vi "Advance past Number.vi"(7 "JSON":string, 9 "Offset (0)":i32, 11 "Parser State in":T2=enum."Number/Other") -> (1 "Offset past match":i32, 2 "LabVIEW Extension (NaN, Infinity)":bool, 3 "Parser State":T2, 4 "JSON Value Type":T1, 6 "Value start out":i32)   [LabVIEW 2020, in "JSONtext.lvlib"]
uses:
  <vilib>/JDP Science/JSONtext/JSONtext.lvlib
  <vilib>/JDP Science/JSONtext/Parsing/Parsing State.ctl
  <vilib>/JDP Science/JSONtext/JSON Value Type.ctl
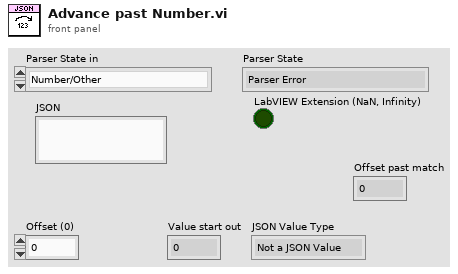
[diagram p1: front panel]
types:
  T1 = typedef "JSONtext.lvlib/JSON Value Type.ctl" = enum16{"Not a JSON Value", "JSON Object", "JSON Array", "String", "Number", "true", "false", "null"}
  T2 = typedef "JSONtext.lvlib/Parsing State.ctl" = enum16{"Parser Error", "Object", "Array", "String", "Number/Other", "Leading Whitespace", "Object end", "Array end", "Value end"}
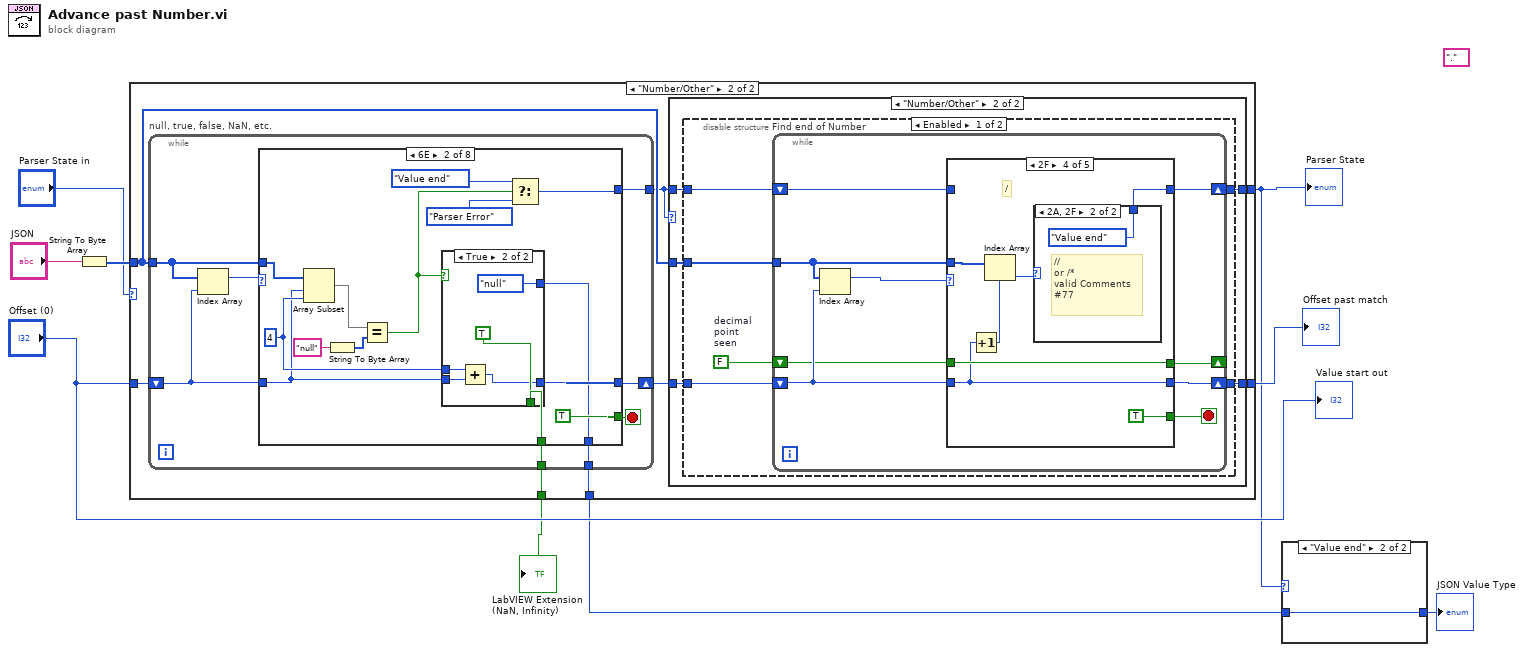
[diagram p0: block diagram]
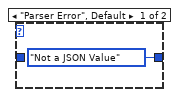
[diagram p2: hidden frame]
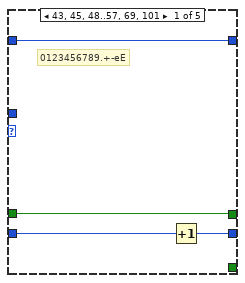
[diagram p5: hidden frame]
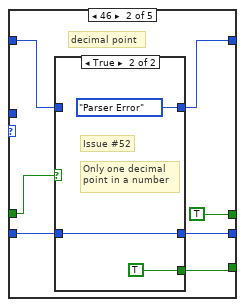
[diagram p6: hidden frame]
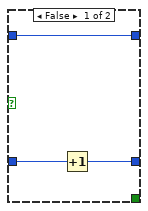
[diagram p7: hidden frame]
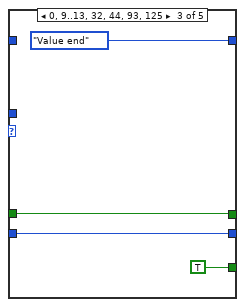
[diagram p8: hidden frame]
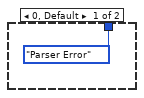
[diagram p9: hidden frame]
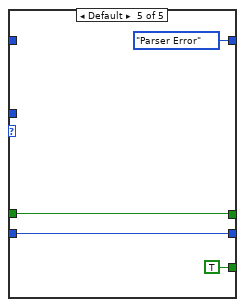
[diagram p10: hidden frame]
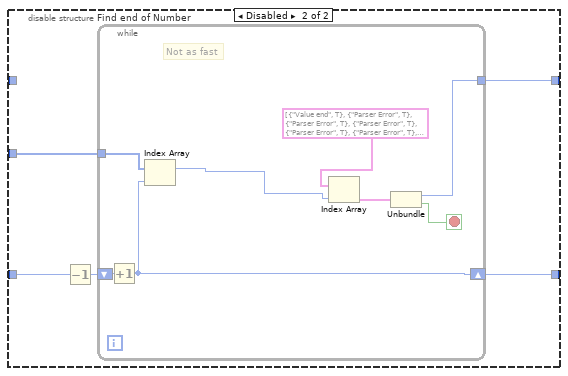
[diagram p11: hidden frame]
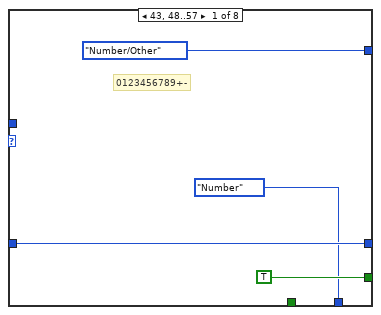
[diagram p12: hidden frame]
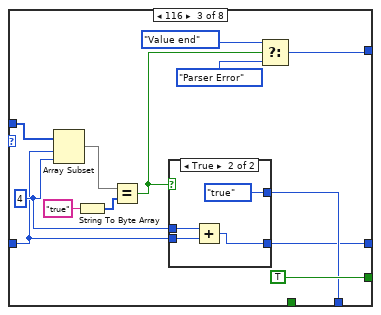
[diagram p14: hidden frame]
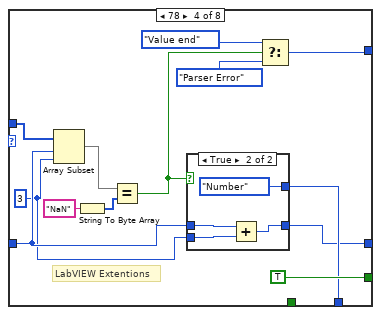
[diagram p16: hidden frame]
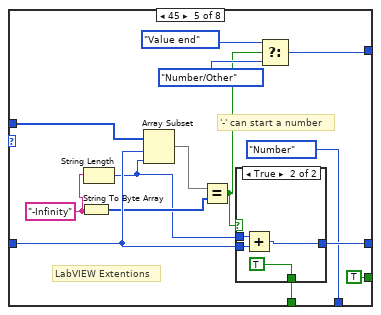
[diagram p18: hidden frame]
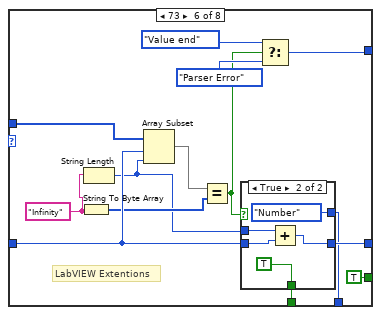
[diagram p20: hidden frame]
diagram:
  (unwired) "."
  n1 = String To Byte Array(string="JSON") -> (unsigned byte array=w6:u8[])
  n2 = case shown="\"Number/Other\"" "Parser State in" {
    tunnel: [_ w18] -> w4
    tunnel: [w10 w17] -> w9
    tunnel: w6 -> [_ w15]
    tunnel: "Offset (0)" -> [w10 w13]
    tunnel: [_ w12] -> w3
    tunnel: [_ w11] -> w1
    frame "Parser Error", Default {
    }
    frame "Number/Other" {
      n3 = while "null, true, false, NaN, etc." {
        tunnel: w15 -> [w94]
        shift-right: [w90] -> w16
        shift-left: w13 -> [w91]
        tunnel: [w93] -> w14
        tunnel: [w89] -> w12
        tunnel: [w88] -> w11
        stop <- w92 stop-if-true
        n4 = Index Array(array=w94, index=w91) -> (element=w95:u8)
        n5 = case shown="6E" w95 {
          tunnel: w94 -> [_ w112 w131 w149 w169 w188 w206 _]
          tunnel: [Parsing_State."Number/Other" w109 w128 w146 w167 w186 w203 Parsing_State."Parser Error"] -> w93
          tunnel: [TRUE TRUE TRUE TRUE TRUE TRUE TRUE TRUE] -> w92
          tunnel: w91 -> [w97 w101 w121 w140 w163 w182 w199 w212]
          tunnel: [w97 w100 w120 w138 w162 w181 w197 w212] -> w90
          tunnel: [JSON_Value_Type."Number" w104 w123 w141 JSON_Value_Type."Number" w176 w195 JSON_Value_Type."Not a JSON Value"] -> w89
          tunnel: [_ w103 _ _ w156 w175 _ _] -> w88
          frame 43, 48..57 {
            # "0123456789+-"
          }
          frame 110 {
            w102 = 4 ("length")
            n6 = Array Subset(array=w112, index=w101, length=w102) -> (w110:u8[])
            n7 = String To Byte Array(string="null") -> (unsigned byte array=w111:u8[])
            n8 = Equal?(x=w110, y=w111) -> (x = y?=w105:bool)
            n9 = case shown="True" w105 {
              tunnel: [_ JSON_Value_Type."null"] -> w104
              tunnel: [_ TRUE] -> w103
              tunnel: w102 -> [_ w117]
              tunnel: w101 -> [w114 w116]
              tunnel: [w114 w115] -> w100
              frame False {
              }
              frame True {
                n10 = Add(x=w117, y=w116) -> (x+y=w115:i32)
              }
            }
            n11 = Select(t=Parsing_State."Value end", s=w105, f=Parsing_State."Parser Error") -> (s? t:f=w109:T2)
          }
          frame 116 {
            w122 = 4 ("length")
            n12 = Array Subset(array=w131, index=w121, length=w122) -> (w129:u8[])
            n13 = String To Byte Array(string="true") -> (unsigned byte array=w130:u8[])
            n14 = Equal?(x=w129, y=w130) -> (x = y?=w124:bool)
            n15 = case shown="True" w124 {
              tunnel: [_ JSON_Value_Type."true"] -> w123
              tunnel: w122 -> [_ w136]
              tunnel: w121 -> [w133 w135]
              tunnel: [w133 w134] -> w120
              frame False {
              }
              frame True {
                n16 = Add(x=w136, y=w135) -> (x+y=w134:i32)
              }
            }
            n17 = Select(t=Parsing_State."Value end", s=w124, f=Parsing_State."Parser Error") -> (s? t:f=w128:T2)
          }
          frame 78 {
            w139 = 3 ("length")
            # "LabVIEW Extentions"
            n18 = Array Subset(array=w149, index=w140, length=w139) -> (w147:u8[])
            n19 = String To Byte Array(string="NaN") -> (unsigned byte array=w148:u8[])
            n20 = Equal?(x=w147, y=w148) -> (x = y?=w142:bool)
            n21 = case shown="True" w142 {
              tunnel: [_ JSON_Value_Type."Number"] -> w141
              tunnel: w140 -> [w151 w154]
              tunnel: w139 -> [_ w153]
              tunnel: [w151 w152] -> w138
              frame False {
              }
              frame True {
                n22 = Add(x=w154, y=w153) -> (x+y=w152:i32)
              }
            }
            n23 = Select(t=Parsing_State."Value end", s=w142, f=Parsing_State."Parser Error") -> (s? t:f=w146:T2)
          }
          frame 45 {
            w160 = "-Infinity"
            # "'-' can start a number"
            # "LabVIEW Extentions"
            n24 = String To Byte Array(string=w160) -> (unsigned byte array=w161:u8[])
            n25 = String Length(string=w160) -> (length=w159:i32)
            n26 = Array Subset(array=w169, index=w163, length=w159) -> (w168:u8[])
            n27 = Equal?(x=w168, y=w161) -> (x = y?=w158:bool)
            n28 = case shown="True" w158 {
              tunnel: w163 -> [w170 w174]
              tunnel: [w170 w173] -> w162
              tunnel: w159 -> [_ w172]
              tunnel: [_ TRUE] -> w156
              frame False {
              }
              frame True {
                n29 = Add(x=w172, y=w174) -> (x+y=w173:i32)
              }
            }
            n30 = Select(t=Parsing_State."Value end", s=w158, f=Parsing_State."Number/Other") -> (s? t:f=w167:T2)
          }
          frame 73 {
            w179 = "Infinity"
            # "LabVIEW Extentions"
            n31 = String To Byte Array(string=w179) -> (unsigned byte array=w180:u8[])
            n32 = String Length(string=w179) -> (length=w178:i32)
            n33 = Array Subset(array=w188, index=w182, length=w178) -> (w187:u8[])
            n34 = Equal?(x=w187, y=w180) -> (x = y?=w177:bool)
            n35 = case shown="True" w177 {
              tunnel: w182 -> [w189 w194]
              tunnel: [w189 w193] -> w181
              tunnel: w178 -> [_ w192]
              tunnel: [_ JSON_Value_Type."Number"] -> w176
              tunnel: [_ TRUE] -> w175
              frame False {
              }
              frame True {
                n36 = Add(x=w192, y=w194) -> (x+y=w193:i32)
              }
            }
            n37 = Select(t=Parsing_State."Value end", s=w177, f=Parsing_State."Parser Error") -> (s? t:f=w186:T2)
          }
          frame 102 {
            w198 = 5 ("length")
            n38 = Array Subset(array=w206, index=w199, length=w198) -> (w204:u8[])
            n39 = String To Byte Array(string="false") -> (unsigned byte array=w205:u8[])
            n40 = Equal?(x=w204, y=w205) -> (x = y?=w196:bool)
            n41 = case shown="True" w196 {
              tunnel: [_ JSON_Value_Type."false"] -> w195
              frame False {
              }
              frame True {
              }
            }
            n42 = Add(x=w198, y=w199) -> (x+y=w197:i32)
            n43 = Select(t=Parsing_State."Value end", s=w196, f=Parsing_State."Parser Error") -> (s? t:f=w203:T2)
          }
          frame Default {
          }
        }
      }
      n44 = case shown="\"Number/Other\"" w14 {
        tunnel: [w19 w25] -> w18
        tunnel: [w20 w24] -> w17
        tunnel: w16 -> [w20 w21]
        tunnel: w14 -> [w19 w23]
        tunnel: w15 -> [_ w22]
        frame "Parser Error", Default {
        }
        frame "Number/Other" {
          n45 = disable-structure shown="Enabled" {
            disable-tunnel: [w31 w79] -> w25
            disable-tunnel: [w30 w78] -> w24
            disable-tunnel: w23 -> [w29 _]
            disable-tunnel: w22 -> [w28 w77]
            disable-tunnel: w21 -> [w27 w76]
            frame Enabled {
              w26 = FALSE  # decimal point seen
              n46 = while "Find end of Number" {
                tunnel: w28 -> [w40]
                shift-right: [w36] -> w30
                shift-left: w27 -> [w34]
                shift-right: [w38] -> w31
                shift-left: w29 -> [w39]
                shift-right: [w33] -> _
                shift-left: w26 -> [w32]
                stop <- w37 stop-if-true
                n47 = Index Array(array=w40, index=w34) -> (element=w35:u8)
                n48 = case shown="2F" w35 {
                  tunnel: w40 -> [_ _ _ w64 _]
                  tunnel: w39 -> [w44 w47 _ _ _]
                  tunnel: [w44 w46 Parsing_State."Value end" w62 Parsing_State."Parser Error"] -> w38
                  tunnel: [_ w45 TRUE TRUE TRUE] -> w37
                  tunnel: w34 -> [w43 w51 w59 w66 w74]
                  tunnel: [w42 w50 w59 w66 w74] -> w36
                  tunnel: [w41 TRUE w58 w67 w71] -> w33
                  tunnel: w32 -> [w41 w48 w58 w67 w71]
                  frame 43, 45, 48..57, 69, 101 {
                    # "0123456789.+-eE"
                    n49 = Increment(x=w43) -> (x+1=w42:i32)
                  }
                  frame 46 {
                    # "decimal point"
                    n50 = case shown="True" w48 {
                      tunnel: w51 -> [w54 w56]
                      tunnel: [w53 w56] -> w50
                      tunnel: [w52 Parsing_State."Parser Error"] -> w46
                      tunnel: w47 -> [w52 _]
                      tunnel: [_ TRUE] -> w45
                      frame False {
                        n51 = Increment(x=w54) -> (x+1=w53:i32)
                      }
                      frame True {
                        # "Only one decimal\npoint in a number"
                        # "Issue #52"
                      }
                    }
                  }
                  frame 0, 9..13, 32, 44, 93, 125 {
                  }
                  frame 47 {
                    # "/"
                    n52 = Increment(x=w66) -> (x+1=w65:i32)
                    n53 = Index Array(array=w64, index=w65) -> (element=w63:u8)
                    n54 = case shown="2A, 2F" w63 {
                      tunnel: [Parsing_State."Parser Error" Parsing_State."Value end"] -> w62
                      frame 0, Default {
                      }
                      frame 42, 47 {
                        # "//\nor /*\nvalid Comments\n#77"
                      }
                    }
                  }
                  frame Default {
                  }
                }
              }
            }
            frame Disabled {
              n55 = Decrement(x=w76) -> (x-1=w75:i32)
              n56 = while "Find end of Number" {
                tunnel: w77 -> [w87]
                shift-right: [w80] -> w78
                shift-left: w75 -> [w86]
                tunnel: [w81] -> w79
                stop <- w82 stop-if-true
                # "Not as fast"
                n57 = Increment(x=w86) -> (x+1=w80:i32)
                n58 = Index Array(array=w87, index=w80) -> (element=w83:u8)
                n59 = Index Array(array=cluster{T2, bool}[] [{enum."Value end", TRUE}, {enum."Parser Error", TRUE}, {enum."Parser Error", TRUE}, {enum."Parser Error", TRUE}, {enum."Parser Error", TRUE}, {enum."Parser Error", TRUE}, {enum."Parser Error", TRUE}, {enum."Parser Error", TRUE}, {enum."Parser Error", TRUE}, {enum."Value end", TRUE}, {enum."Value end", TRUE}, {enum."Value end", TRUE}, {enum."Value end", TRUE}, {enum."Value end", TRUE}, {enum."Parser Error", TRUE}, {enum."Parser Error", TRUE}, {enum."Parser Error", TRUE}, {enum."Parser Error", TRUE}, {enum."Parser Error", TRUE}, {enum."Parser Error", TRUE}, {enum."Parser Error", TRUE}, {enum."Parser Error", TRUE}, {enum."Parser Error", TRUE}, {enum."Parser Error", TRUE}, {enum."Parser Error", TRUE}, {enum."Parser Error", TRUE}, {enum."Parser Error", TRUE}, {enum."Parser Error", TRUE}, {enum."Parser Error", TRUE}, {enum."Parser Error", TRUE}, {enum."Parser Error", TRUE}, {enum."Parser Error", TRUE}, {enum."Value end", TRUE}, {enum."Parser Error", TRUE}, {enum."Parser Error", TRUE}, {enum."Parser Error", TRUE}, {enum."Parser Error", TRUE}, {enum."Parser Error", TRUE}, {enum."Parser Error", TRUE}, {enum."Parser Error", TRUE}, {enum."Parser Error", TRUE}, {enum."Parser Error", TRUE}, {enum."Parser Error", TRUE}, {enum."Number/Other", FALSE}, {enum."Value end", TRUE}, {enum."Number/Other", FALSE}, {enum."Number/Other", FALSE}, {enum."Parser Error", TRUE}, {enum."Number/Other", FALSE}, {enum."Number/Other", FALSE}, {enum."Number/Other", FALSE}, {enum."Number/Other", FALSE}, {enum."Number/Other", FALSE}, {enum."Number/Other", FALSE}, {enum."Number/Other", FALSE}, {enum."Number/Other", FALSE}, {enum."Number/Other", FALSE}, {enum."Number/Other", FALSE}, {enum."Parser Error", TRUE}, {enum."Parser Error", TRUE}, {enum."Parser Error", TRUE}, {enum."Parser Error", TRUE}, {enum."Parser Error", TRUE}, {enum."Parser Error", TRUE}, {enum."Parser Error", TRUE}, {enum."Parser Error", TRUE}, {enum."Parser Error", TRUE}, {enum."Parser Error", TRUE}, {enum."Parser Error", TRUE}, {enum."Number/Other", FALSE}, {enum."Parser Error", TRUE}, {enum."Parser Error", TRUE}, {enum."Parser Error", TRUE}, {enum."Parser Error", TRUE}, {enum."Parser Error", TRUE}, {enum."Parser Error", TRUE}, {enum."Parser Error", TRUE}, {enum."Parser Error", TRUE}, {enum."Parser Error", TRUE}, {enum."Parser Error", TRUE}, {enum."Parser Error", TRUE}, {enum."Parser Error", TRUE}, {enum."Parser Error", TRUE}, {enum."Parser Error", TRUE}, {enum."Parser Error", TRUE}, {enum."Parser Error", TRUE}, {enum."Parser Error", TRUE}, {enum."Parser Error", TRUE}, {enum."Parser Error", TRUE}, {enum."Parser Error", TRUE}, {enum."Parser Error", TRUE}, {enum."Parser Error", TRUE}, {enum."Parser Error", TRUE}, {enum."Value end", TRUE}, {enum."Parser Error", TRUE}, {enum."Parser Error", TRUE}, {enum."Parser Error", TRUE}, {enum."Parser Error", TRUE}, {enum."Parser Error", TRUE}, {enum."Parser Error", TRUE}, {enum."Parser Error", TRUE}, {enum."Number/Other", FALSE}, {enum."Parser Error", TRUE}, {enum."Parser Error", TRUE}, {enum."Parser Error", TRUE}, {enum."Parser Error", TRUE}, {enum."Parser Error", TRUE}, {enum."Parser Error", TRUE}, {enum."Parser Error", TRUE}, {enum."Parser Error", TRUE}, {enum."Parser Error", TRUE}, {enum."Parser Error", TRUE}, {enum."Parser Error", TRUE}, {enum."Parser Error", TRUE}, {enum."Parser Error", TRUE}, {enum."Parser Error", TRUE}, {enum."Parser Error", TRUE}, {enum."Parser Error", TRUE}, {enum."Parser Error", TRUE}, {enum."Parser Error", TRUE}, {enum."Parser Error", TRUE}, {enum."Parser Error", TRUE}, {enum."Parser Error", TRUE}, {enum."Parser Error", TRUE}, {enum."Parser Error", TRUE}, {enum."Value end", TRUE}] ("Array"), index=w83) -> (element=w84:cluster{T2, bool})
                n60 = Unbundle(w84) -> (w81:T2, w82:bool)
              }
            }
          }
        }
      }
    }
  }
  "Parser State" <- w4
  "Offset past match" <- w9
  "LabVIEW Extension (NaN, Infinity)" <- w1
  n61 = case shown="\"Value end\"" w4 {
    tunnel: w3 -> [_ w214]
    tunnel: [JSON_Value_Type."Not a JSON Value" w214] -> w2
    frame "Parser Error", Default {
    }
    frame "Value end" {
    }
  }
  "JSON Value Type" <- w2
  "Value start out" <- "Offset (0)"
